vi "Add Item.vi"(8 "error in (no error)":errorcluster, 10 "Item":T1, 11 "Monkey in":refnum<class "Monkey.lvclass">) -> (0 "error out":errorcluster, 3 "Monkey out":refnum<class "Monkey.lvclass">)   [LabVIEW 2022 SP3, in "AoC22.lvlib" / "Monkey.lvclass"]
uses:
  Monkey.lvclass
  Monkey.lvclass/Monkey.ctl
  Worry Level.ctl
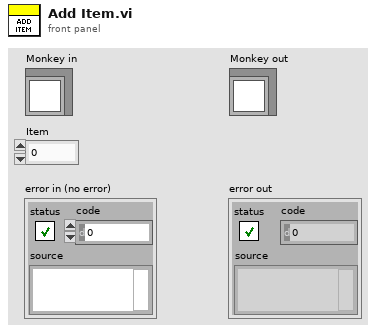
[diagram p1: front panel]
types:
  T1 = typedef "AoC22.lvlib/Monkey.lvclass/Worry Level.ctl" = ext
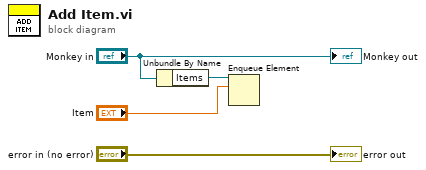
[diagram p0: block diagram]
diagram:
  n1 = Unbundle By Name("Monkey in") -> ("Items"=w2:refnum<queue>)
  n2 = Enqueue Element(queue=w2, element="Item") -> ()  [unwired: 2 in, 3 out]
  "error out" <- "error in (no error)"
  "Monkey out" <- "Monkey in"
